vi "Error-Query.vi"(8 "error in (no error)":errorcluster {"code" format="%.0x"}, 11 "instrument handle":refnum<k15>) -> (0 "error out":errorcluster {"code" format="%.0x"}, 1 "error message":string, 2 "error code":i32 format="%.0g", 3 "instrument handle out":refnum<k15>)   [LabVIEW 2014, in "Agilent NA.lvlib"]
doc: "Queries the instrument and returns instrument specific error information. This VI can be used when QueryInstrumentStatus is True to retrieve error details when the driver detects an instrument error."
uses:
  Agilent NA.lvlib
  AgNA.dll
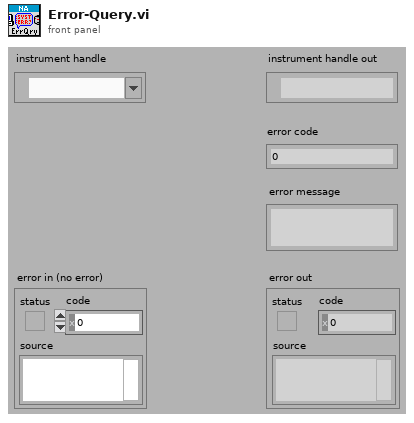
[diagram p1: front panel]
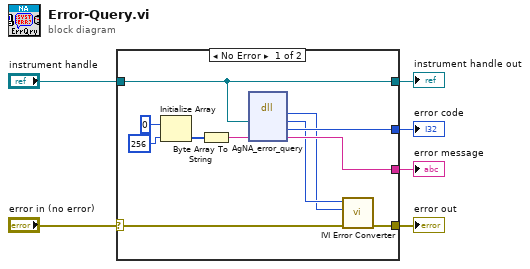
[diagram p0: block diagram]
diagram:
  n1 = case shown="No Error" "error in (no error)" {
    selector: "error in (no error)" -> [w8 w18]
    tunnel: "instrument handle" -> [w7 w19]
    tunnel: [w14 _] -> w5
    tunnel: [w12 _] -> w4
    tunnel: [w10 w18] -> w3
    tunnel: [w7 w19] -> w1
    frame No Error {
      n2 = Initialize Array(u8 0, 256) -> (w15:u8[])
      n3 = Byte Array To String(unsigned byte array=w15) -> (string=w13:string)
      n4 = dll-call lib="AgNA**.dll" fn="AgNA_error_query" ("LabVIEW:IviDmm_error_query")("instrument handle"=w7, "error message"=w13) -> ("Status"=w9:i32, "instrument handle"=w11:u32, "error code"=w14:i32, "error message"=w12:string)  [unwired: 3 in, 3 out]
      n5 = call "IVI Error Converter.vi"("error in (no error)"=w8, "IVI error code (0)"=w9, "instrument handle"=w11) -> ("error out"=w10:errorcluster)  [unwired: 7 in, 1 out]
    }
    frame Error {
    }
  }
  "instrument handle out" <- w1
  "error code" <- w5
  "error message" <- w4
  "error out" <- w3
